vi "Set Elevator Position from Location.vi"(8 "error in (no error)":errorcluster, 10 "Elevator Position":u8(slide) scale=1.0..4.0, 11 "Elevator Controller Actor in":refnum<class "Elevator Controller Actor.lvclass">) -> (0 "error out":errorcluster, 3 "Elevator Controller Actor out":refnum<class "Elevator Controller Actor.lvclass">)   [LabVIEW 2019]
uses:
  Simulated Sensor Interface Actor/Sim Sensor Interface Messages/Update Elevator Position Msg/Update Elevator Position Msg.lvclass
  Elevator Controller Actor.lvclass
  C:/Program Files (x86)/National Instruments/LabVIEW 2019/vi.lib/ActorFramework/Actor/Actor.lvclass
  <vilib>/ActorFramework/Message Enqueuer/Message Enqueuer.lvclass
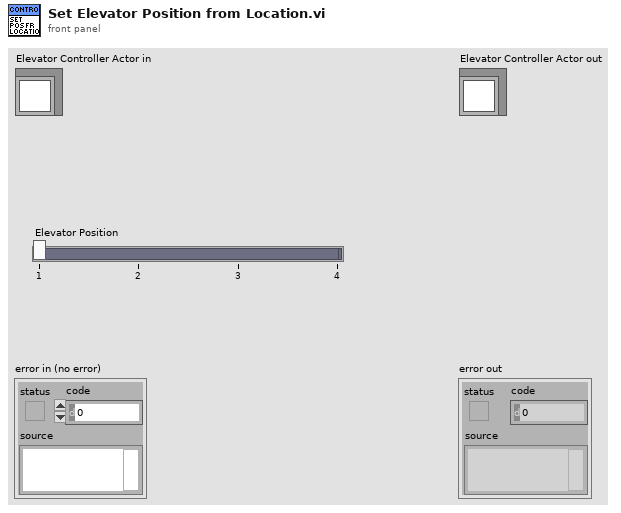
[diagram p1: front panel]
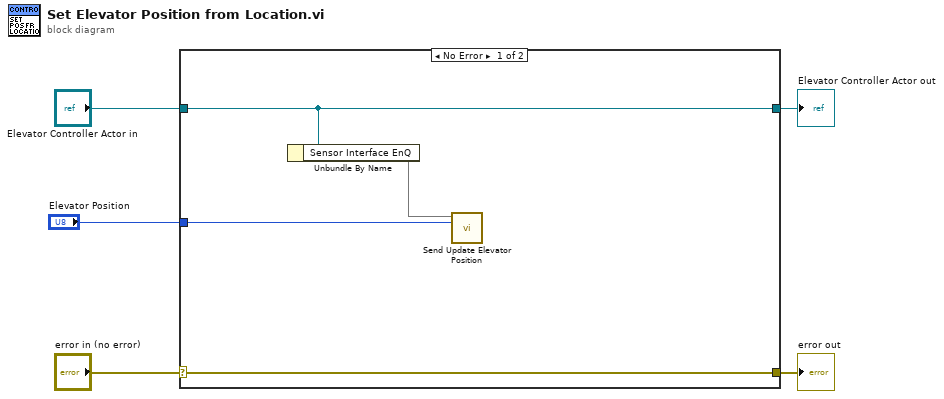
[diagram p0: block diagram]
diagram:
  n1 = case shown="No Error" "error in (no error)" {
    selector: "error in (no error)" -> [w9 w11]
    tunnel: [w9 w11] -> w4
    tunnel: [w8 w10] -> w2
    tunnel: "Elevator Controller Actor in" -> [w8 w10]
    tunnel: "Elevator Position" -> [w6 _]
    frame No Error {
      n2 = Unbundle By Name(w8) -> ("Sensor Interface EnQ"=w7)
      n3 = call "Send Update Elevator Position.vi"("Elevator Position"=w6, "Message Enqueuer"=w7) -> ()  [unwired: 8 in, 2 out]
    }
    frame Error {
    }
  }
  "error out" <- w4
  "Elevator Controller Actor out" <- w2
